vi "Read Rooms.vi"(8 "error in (no error)":errorcluster, 11 "State Key in":refnum<class "State Key.lvclass">) -> (0 "error out":errorcluster, 2 "Rooms":string[][](array[string]), 3 "State Key out":refnum<class "State Key.lvclass">)   [LabVIEW 2019, in "23.lvlib" / "State Key.lvclass"]
uses:
  State Key.lvclass
  State Key.lvclass/State Key.ctl
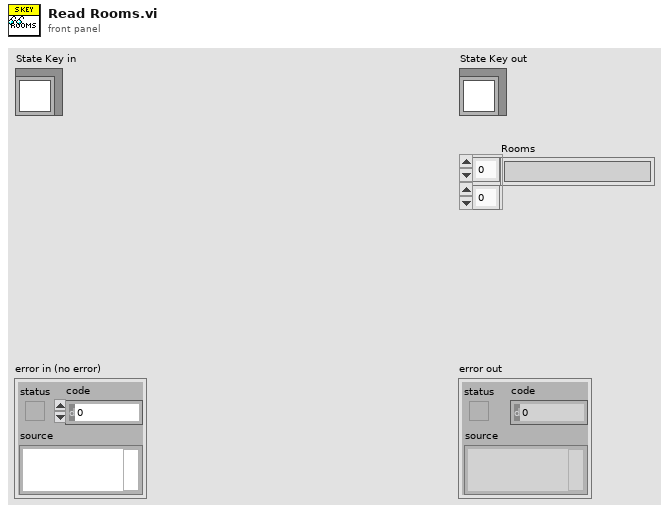
[diagram p1: front panel]
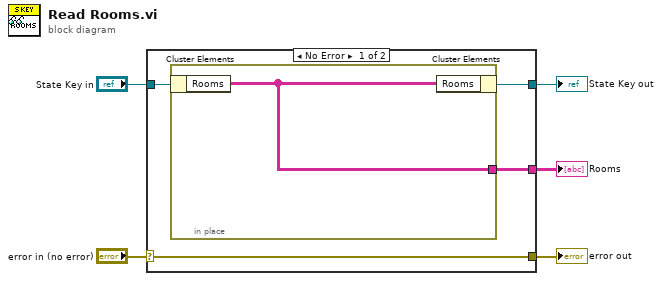
[diagram p0: block diagram]
diagram:
  n1 = case shown="No Error" "error in (no error)" {
    selector: "error in (no error)" -> [w9 w11]
    tunnel: [w9 w11] -> w4
    tunnel: [w6 w12] -> w2
    tunnel: "State Key in" -> [w7 w12]
    tunnel: [w8 _] -> w1
    frame No Error {
      n2 = in-place {
        in-place-border: [w10] -> w8
        n3 = in-place-cluster #1(w7) -> ("Rooms"=w10:string[][])
        n4 = in-place-cluster #1("Rooms"=w10) -> (w6:refnum<class "State Key.lvclass">)
      }
    }
    frame Error {
    }
  }
  "error out" <- w4
  "State Key out" <- w2
  "Rooms" <- w1
